vi "golpi_mpc_init_session.vi"(8 "error in":errorcluster, 11 "golpi session in":T1={"GOLPI ref"={"pipe handle"={"lv_proc.dll file path"=path "", "process instance handle"=[], "debug mode"=FALSE, "debug data"=[]}, "fast read timeout [ms]"=500, "fast read settle time [ms]"=10, "fast read to multiple [ms]"=1, "max elements per input line"=100, "slow read timeout [ms]"=5000, "stdin double format specifier"="%_16e", "max elements per stdout output column"=100, "console mode bitstream"=FALSE, "bitstream first read timeout [ms]"=1000, "bitstream read timeout [ms]"=50, "struct transfer possible"=FALSE, "matlab mode"=FALSE}, "idn str"="", "octave path"=path "C:/Octave364/Octave3.6.4_gcc4.6.2/bin", "work path"=path "C:/Octave364/Octave3.6.4_gcc4.6.2/bin", "start timeout [ms]"=15000, "clr cache"=FALSE, "console"=FALSE, "binary"=FALSE, "semaphore"=refnum, "initial command"="", "exit command"="", "matlab"=FALSE}) -> (0 "error out":errorcluster, 3 "golpi session out":T1={"GOLPI ref"={"pipe handle"={"lv_proc.dll file path"=path "", "process instance handle"=[], "debug mode"=FALSE, "debug data"=[]}, "fast read timeout [ms]"=500, "fast read settle time [ms]"=10, "fast read to multiple [ms]"=1, "max elements per input line"=100, "slow read timeout [ms]"=5000, "stdin double format specifier"="%_16e", "max elements per stdout output column"=100, "console mode bitstream"=FALSE, "bitstream first read timeout [ms]"=1000, "bitstream read timeout [ms]"=50, "struct transfer possible"=FALSE, "matlab mode"=FALSE}, "idn str"="", "octave path"=path "C:/Octave364/Octave3.6.4_gcc4.6.2/bin", "work path"=path "C:/Octave364/Octave3.6.4_gcc4.6.2/bin", "start timeout [ms]"=15000, "clr cache"=FALSE, "console"=FALSE, "binary"=FALSE, "semaphore"=refnum, "initial command"="", "exit command"="", "matlab"=FALSE})   [LabVIEW 2018, in "GOLPI Multi Process.lvlib"]
doc: "Initialization of GOLPI multi-process unit. Call this before using any other multi-process communication with GOLPI. It creates semaphore which is later used for exclusive access to the GOLPI to prevent race condition.\n\nNote: This is the only function from GOLPI multi-process unit that assecces the GOLPI session variable directly because it is intended to be placed in the main VI where the session variable is located. Put all setting into the session clusted before calling this VI. Then call it, and then do not access the session variable directly anymore otherwise race condition may occure! All other VIs from this unit accessed the variable indirectly via reference."
uses:
  GOLPI Multi Process.lvlib
  golpi_session.ctl
  GOLPI Library.lvlibp/Public/GOLPI reference Type Def.ctl
  GOLPI Library.lvlibp/LV Process source distribution/Pipe Handle.ctl
  GOLPI Library.lvlibp/LV Process source distribution/LV Process library.lvlib
  GOLPI Library.lvlibp
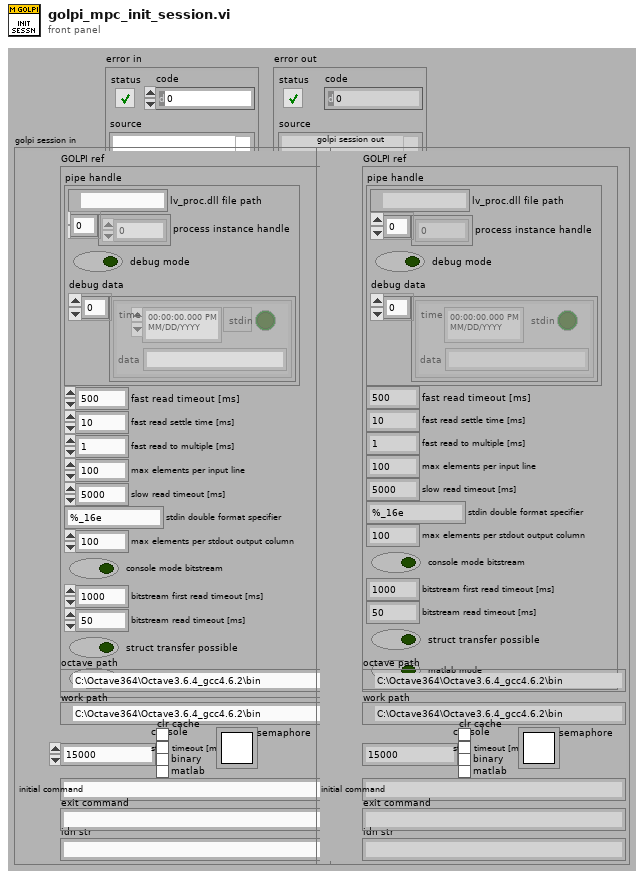
[diagram p1: front panel]
types:
  T1 = typedef "GOLPI Multi Process.lvlib/golpi_session.ctl" = cluster{"GOLPI ref":T2, "idn str":string, "octave path":path, "work path":path, "start timeout [ms]":u32, "clr cache":bool, "console":bool, "binary":bool, "semaphore":T4, "initial command":string, "exit command":string, "matlab":bool}
  T2 = typedef "GOLPI Library.lvlibp/GOLPI reference Type Def.ctl" = cluster{"pipe handle":T3, "fast read timeout [ms]":u32, "fast read settle time [ms]":u32, "fast read to multiple [ms]":u32, "max elements per input line":u32, "slow read timeout [ms]":u32, "stdin double format specifier":string, "max elements per stdout output column":u32, "console mode bitstream":bool, "bitstream first read timeout [ms]":u32, "bitstream read timeout [ms]":u32, "struct transfer possible":bool, "matlab mode":bool}
  T3 = typedef "GOLPI Library.lvlibp/LV Process library.lvlib/Pipe Handle.ctl" = cluster{"lv_proc.dll file path":path, "process instance handle":u32[], "debug mode":bool, "debug data":cluster{"time":timestamp, "stdin":bool, "data":string}[]}
  T4 = typedef "Semaphore RefNum" = refnum<k1>
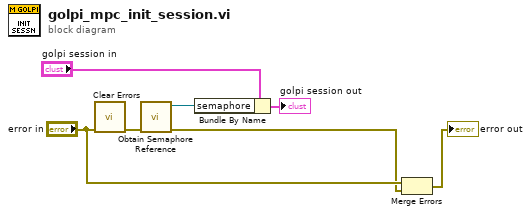
[diagram p0: block diagram]
diagram:
  n1 = call <vilib>:"Clear Errors.vi"("error in (no error)"="error in") -> ("error out"=w6:errorcluster)  [unwired: 5 in, 1 out]
  n2 = call <vilib>:"Obtain Semaphore Reference.vi"("error in (no error)"=w6) -> ("error out"=w2:errorcluster, "semaphore"=w7:T4)  [unwired: 4 in, 1 out]
  n3 = Bundle By Name(cluster="golpi session in", "semaphore"=w7) -> (→"golpi session out":T1)
  n4 = Merge Errors("error in", w2) -> (→"error out":errorcluster)
